vi "Dashboard Main bad.vi"() -> ()   [LabVIEW 2012]
uses:
  <vilib>/event_ctls.llb/eventvkey.ctl
  <vilib>/Utility/config.llb/Read Key (String).vi
  <vilib>/Utility/config.llb/Read Key (I32).vi
  <vilib>/Utility/config.llb/Write Key (String).vi
  <vilib>/Utility/config.llb/Write Key (I32).vi
  Program Files (x86)/National Instruments/LabVIEW 2012/examples/FRC/Vision/Rectangular Target - 2013/Robot Global Data.vi
  <vilib>/Utility/config.llb/NI_LVConfig.lvlib
  <vilib>/vision/NI_Vision_Development_Module.lvlib
  <vilib>/gmath/NI_Gmath.lvlib
panel:
  out "mean red":dbl
  out "mean blue":dbl
  out "mean green":dbl
  out "max red":dbl
  out "min red":dbl
  out "max blue":dbl
  out "min blue":dbl
  out "max green":dbl
  out "min green":dbl
  in  "Margins":cluster{"Hue":i32, "Sat":i32, "Val":i32}={"Hue"=33, "Sat"=53, "Val"=9} {"Sat" scale=0.0..80.0; "Val" scale=0.0..80.0; "Hue" scale=0.0..80.0}
  in  "Hue 2":i32(knob)=65 scale=0.0..255.0
  in  "Saturation 2":i32=255
  in  "Luminance":i32=255
  out "Hue":cluster{i32, i32}
  out "Saturation":cluster{i32, i32}
  out "Value":cluster{i32, i32}
  out "Target Info":T1(array[cluster])
  in  "Score Limits":T2={"Rect Coverage"=60.0, "X Edge Strength"=40.0, "Y Edge Strength"=60.0, "Center"=75.0, "Outer"=75.0}
  in  "Area Size Limit %":dbl=0.5
  in  "Particle Count Limit":i32=8
  out "Battery Value":dbl(slide) scale=0.0..14.0 scale format="%#_2e"
  out "Battery":sgl(graph)
  in  "Camera Settings":T3={"Frate Rate"=30, "Compression"=30, "Size"=1} {"Frate Rate" scale=1.0..30.0; "Size" items=["640x480", "320x240", "160x120"]}
  out "Mode":T4(ring)=enum."Auto Disabled"
  out "Camera IP":string
  out "JS1 Z":dbl(slide) scale=-1.0..1.0 scale format="%#_2e"
  out "JS2 Z":dbl(slide) scale=-1.0..1.0 scale format="%#_2e"
  out "Joystick 1":cluster{"X":dbl, "Y":dbl}[](graph)
  out "Joystick 2":cluster{"X":dbl, "Y":dbl}[](graph)
  out "JS Buttons 1":T5
  out "JS Buttons 2":T5
  out "MotorSlide4":dbl(slide) scale=-1.0..1.0 scale format="%#_2e"
  out "MotorSlide3":dbl(slide) scale=-1.0..1.0 scale format="%#_2e"
  out "MotorSlide2":dbl(slide) scale=-1.0..1.0 scale format="%#_2e"
  in  "MotorName3":string="Front Left"
  in  "MotorName4":string="Front Right"
  in  "MotorName1":string="Rear Left"
  in  "MotorName2":string="Rear Right"
  out "MotorChart4":dbl(graph)
  out "MotorChart3":dbl(graph)
  out "MotorChart2":dbl(graph)
  out "MotorSlide1":dbl(slide) scale=-1.0..1.0 scale format="%#_2e"
  out "MotorChart1":dbl(graph)
  out "Robot IP":string
  in  "Dashboard Tab":enum32{"Operation", "Test", "Checklist"}(tab)
  in  "Checkbox 2":bool
  in  "Checkbox 1":bool
  in  "Slider 1":dbl(slide) scale=0.0..100.0
  in  "Slider":dbl(slide) scale=0.0..100.0 scale format="%#_3g"
  in  "On/Off":bool caption="Solenoid"
  in  "Test Name":u16(ring) items=["Select the test to run...", "Example Test", "-------------------------------", "List of tests is built in robot code.", "Replace with your own automated tests."]
  in  "Test Tree":string(tree)
  in  "Motor":cluster{"Value":dbl, "Enable":bool} {"Value" scale=-1.0..1.0 scale format="%#_3g"}
  out "Progress":T6 {"Test Progress" scale=0.0..100.0}
  in  "Rev/Fwd":cluster{"Forward":bool, "Reverse":bool}
  in  "Ring":u16(ring) items=["Auto", "Fixed indoor", "Fixed outdoor 1", "Fixed outdoor 2", "Fixed fluorescent 1", "Fixed fluorescent 2", "Hold current"]
  in  "Listbox":i32(listbox)
  in  "Viewer":T7(tab)
  out "Mbps":dbl format="%#.1g"
  in  "Enable":bool=TRUE
  in  "DB Camera Config":bool
  out "Mbps":bool
  out "fps":dbl format="%#.1g"
  out "Image Error Message":string="Timeout in Camera Communications"
  out "Original Image":T8(plugin-control)
  in  "View":bool=TRUE
  out "Processed Image":T8(plugin-control)
  in  "View 2":bool=TRUE
  out "Tree":string(tree)
  # "Drive & Motors"
  # "Robot IP:"
  # "Customize by placing controls and indicators here and name to match\nDashboard Variables on robot."
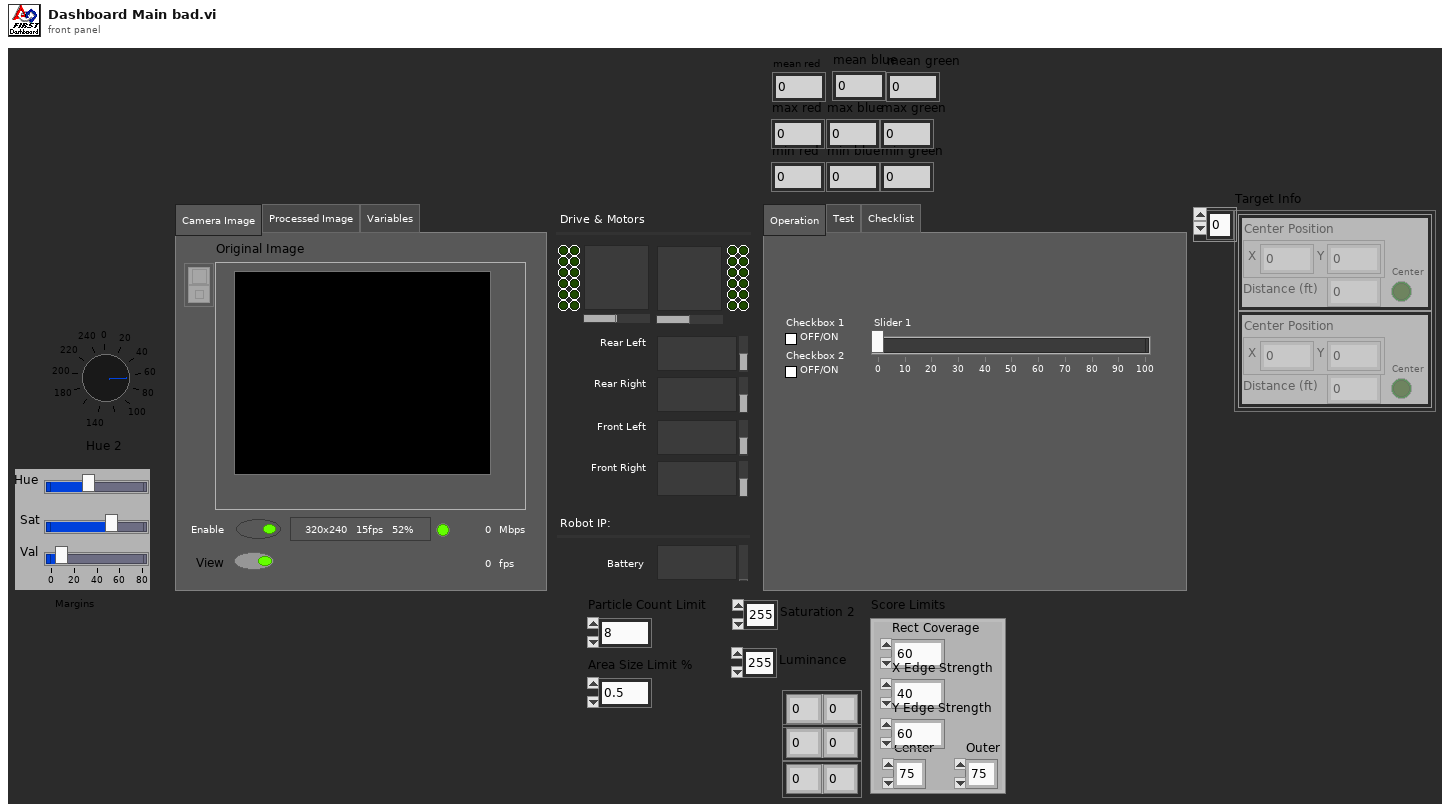
[diagram p1: front panel]
types:
  T1 = cluster{"Center Position":cluster{"X":dbl, "Y":dbl}, "Distance (ft)":dbl, "Center":bool}[]
  T2 = cluster{"Rect Coverage":dbl, "X Edge Strength":dbl, "Y Edge Strength":dbl, "Center":dbl, "Outer":dbl}
  T3 = cluster{"Frate Rate":i32, "Compression":i32, "Size":u16}
  T4 = enum8{"Tele-Op Disabled", "Tele-Op Enabled", "Auto Disabled", "Auto Enabled", "Test Disabled", "Test Enabled", ""}
  T5 = cluster{bool, bool, bool, bool, bool, bool, bool, bool, bool, bool, bool, bool}
  T6 = cluster{"Test Progress":u8, "Test Progress Text":string}
  T7 = enum32{"Camera Image", "Processed Image", "Variables"}
  T8 = typedef "IMAQ Image.ctl" = refnum<image>
  T9 = typedef "Image Type" = u32
  T10 = typedef "LVRectTypeDef.ctl" = cluster{"Left":i16, "Top":i16, "Right":i16, "Bottom":i16}
  T11 = cluster{"Left":i16, "Top":i16, "Right":i16, "Bottom":i16}
  T12 = cluster{"Competition mode":bool, "Robot Link":bool, "Autonomous":bool, "Enabled":bool, "E-Stop":bool, "Simulated":bool, "TestMode":bool, "Docked Window":bool}
  T13 = cluster{"Boolean Array[0]":bool, "Boolean Array[1]":bool, "Boolean Array[2]":bool, "Boolean Array[3]":bool, "Boolean Array[4]":bool, "Boolean Array[5]":bool, "Boolean Array[6]":bool, "Boolean Array[7]":bool, "Boolean Array[8]":bool, "Boolean Array[9]":bool, "Boolean Array[10]":bool, "Boolean Array[11]":bool}
  T14 = cluster{"Position":cluster{"X":dbl, "Y":dbl}, "Distance (ft)":dbl, "Center":bool}[]
  T15 = enum16{"arithmetic", "geometric", "harmonic", "trimmed", "median"}
  T16 = cluster{cluster{"Left":dbl, "Top":dbl, "Right":dbl, "Bottom":dbl}, "Scores":dbl[], cluster{"Long":dbl, "Short":dbl}}[]
  T17 = cluster{"Target Center (-1 to 1)":cluster{"X":dbl, "Y":dbl}, "Distance (ft)":dbl, "Center Target":bool}
  T18 = cluster{"Target Center (-1 to 1)":cluster{"X":dbl, "Y":dbl}, "Distance (ft)":dbl, "Center Target":bool}[]
  T19 = cluster{"Left":dbl, "Top":dbl, "Right":dbl, "Bottom":dbl}
  T20 = typedef "NI_LVConfig.lvlib/Config Data RefNum.ctl" = refnum<k1>
  T21 = typedef "eventvkey.ctl" = enum16{"ASCII", "Enter", "Return", "Shift", "Ctrl", "Alt", "Cmd", "Opt", "Caps", "NumLock", "Clear", "Break", "Up", "Down", "Left", "Right", "Insert", "Delete", "Home", "End", "PageUp", "PageDown", "Escape", "Help", "Pause", "ScrollLock", "F1", "F2", "F3", "F4", "F5", "F6", "F7", "F8", "F9", "F10", "F11", "F12", "F13", "F14", "F15", "F16", "F17", "F18", "F19", "F20", "F21", "F22", "F23", "F24", "Play", "VolumeUp", "VolumeDown", "Mute", "Two Byte Char"}
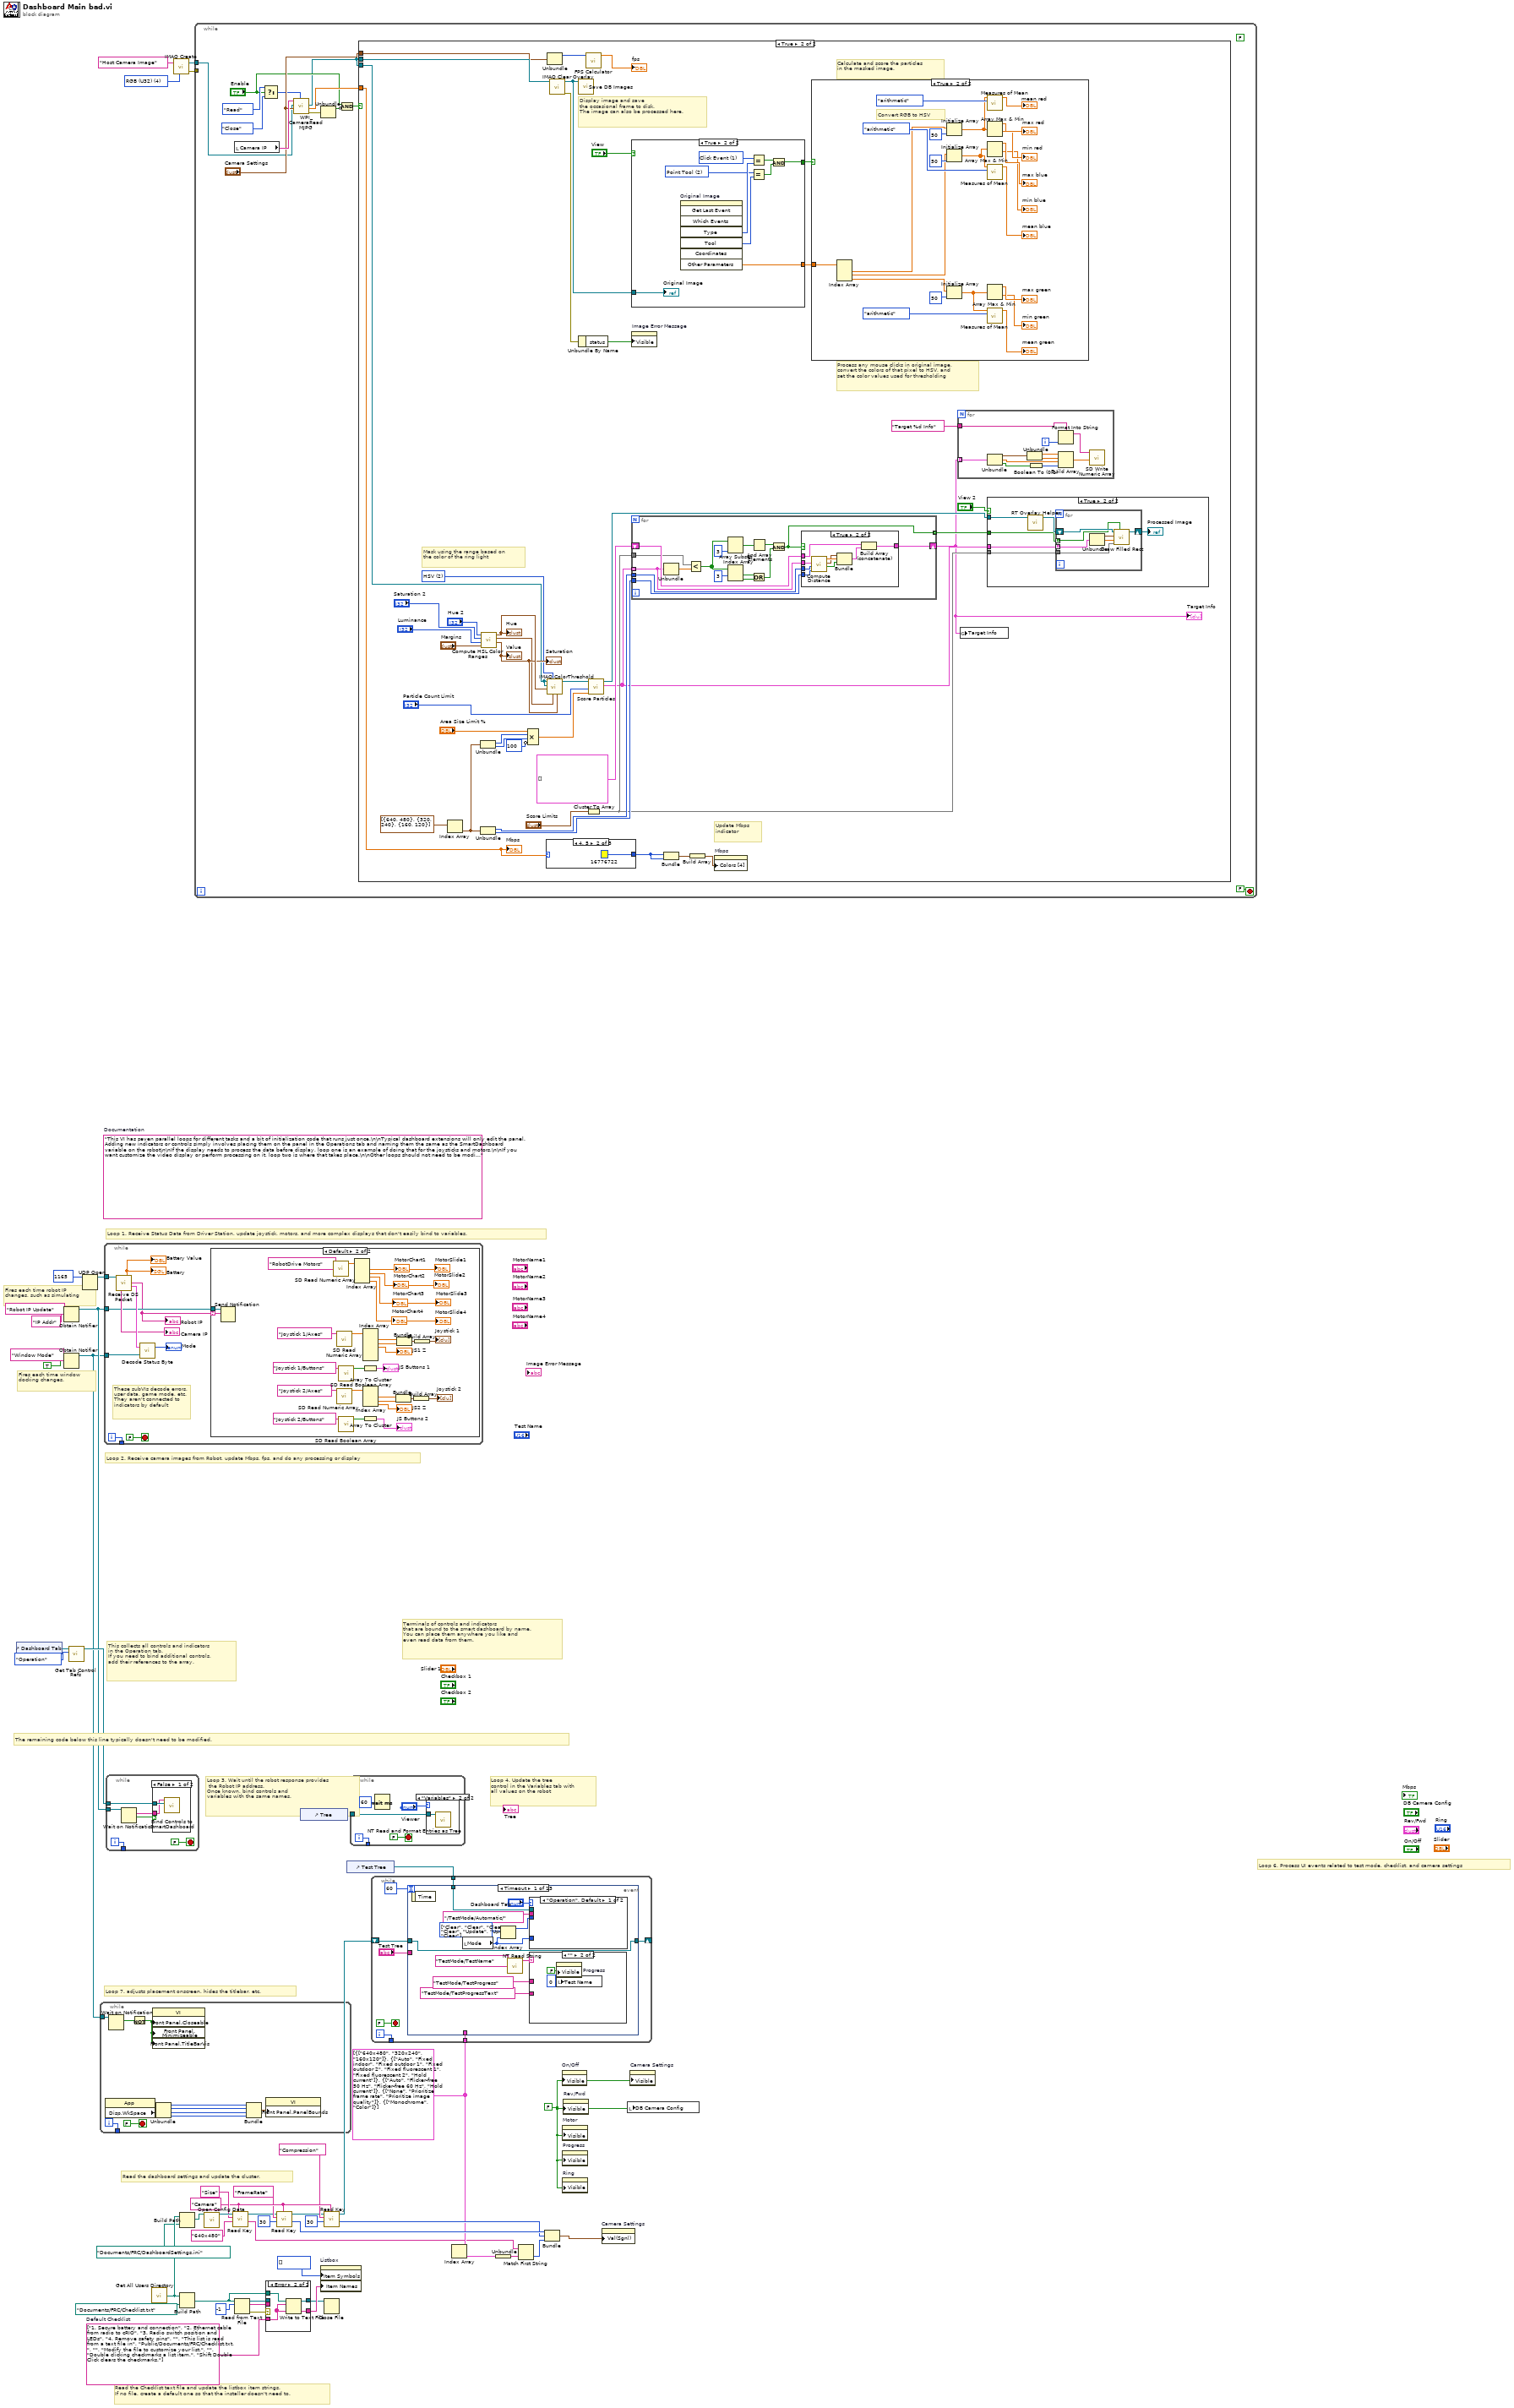
[diagram p0: block diagram]
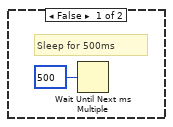
[diagram p3: hidden frame]
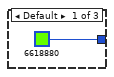
[diagram p8: hidden frame]
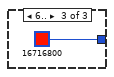
[diagram p9: hidden frame]
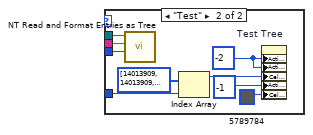
[diagram p11: hidden frame]
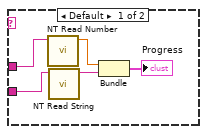
[diagram p12: hidden frame]
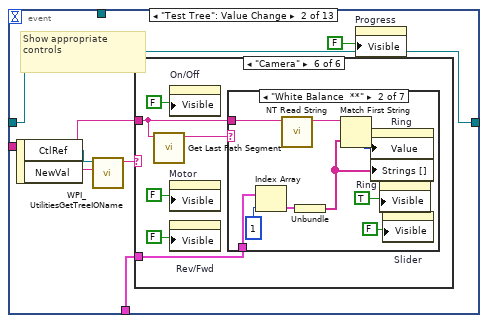
[diagram p13: hidden frame]
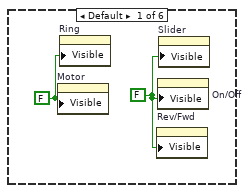
[diagram p14: hidden frame]
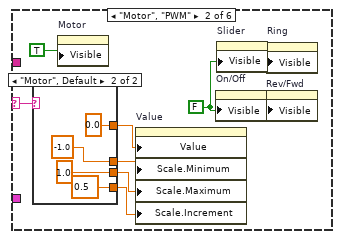
[diagram p15: hidden frame]
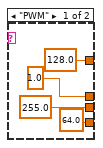
[diagram p16: hidden frame]
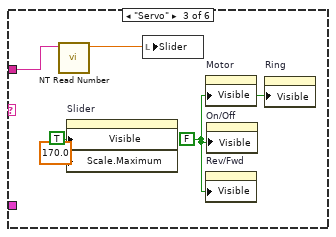
[diagram p17: hidden frame]
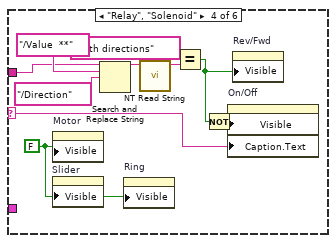
[diagram p18: hidden frame]
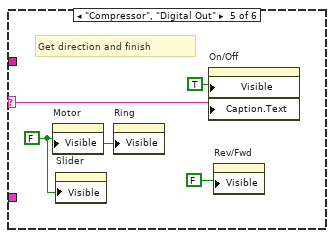
[diagram p19: hidden frame]
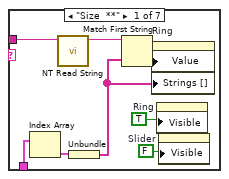
[diagram p20: hidden frame]
diagram:
  w21 = "Camera"
  w13 = cluster{string[]}[] [{["640x480", "320x240", "160x120"]}, {["Auto", "Fixed indoor", "Fixed outdoor 1", "Fixed outdoor 2", "Fixed fluorescent 1", "Fixed fluorescent 2", "Hold current"]}, {["Auto", "Flicker-free 50 Hz", "Flicker-free 60 Hz", "Hold current"]}, {["None", "Prioritize frame rate", "Prioritize image quality"]}, {["Monochrome", "Color"]}]
  w29 = string[] ["1. Secure battery and connection", "2. Ethernet cable from radio to cRIO", "3. Radio switch position and LEDs", "4. Remove safety pins", "", "This list is read from a text file in", "Public/Documents/FRC/Checklist.txt.", "", "Modify the file to customize your list.", "", "Double clicking checkmarks a list item.", "Shift Double Click clears the checkmarks."]  # Default Checklist
  w27 = FALSE ("Visible")
  (unwired) "This VI has seven parallel loops for different tasks and a bit of initialization code that runs just once.\n\nTypical dashboard extensions will only edit the panel. Adding new indicators or controls simply involves placing them on the panel in the Operations tab and naming them the same as the SmartDashboard variable on the robot\n\nIf the display needs to process the data before display, loop one is an example of doing that for the joysticks and motors.\n\nIf you want customize the video display or perform processing on it, loop two is where that takes place.\n\nOther loops should not need to be modified. They are pretty standard, and document the task they perform."  # Documentation
  w48 = T9 4 items=["Grayscale (U8)", "Grayscale (I16)", "Grayscale (SGL)", "Complex (CSG)", "RGB (U32)", "HSL (U32)", "RGB (U64)"] ("Image Type")
  # "Fires each time robot IP\nchanges, such as simulating"
  # "Fires each time window\ndocking changes."
  # "Read the Checklist text file and update the listbox item strings.\nIf no file, create a default one so that the installer doesn't need to."
  # "This collects all controls and indicators\nin the Operation tab.\nIf you need to bind additional controls,\nadd their references to the array."
  # "The remaining code below this line typically doesn't need to be modified."
  # "Loop 6. Process UI events related to test mode, checklist, and camera settings"
  # "Read the dashboard settings and update the cluster."
  # "Terminals of controls and indicators\nthat are bound to the smart dashboard by name.\nYou can place them anywhere you like and\neven read data from them."
  # "Loop 4. Update the tree\ncontrol in the Variables tab with\nall values on the robot"
  # "Loop 3. Wait until the robot response provides\n the Robot IP address.\nOnce known, bind controls and\nvariables with the same names."
  # "Loop 7. adjusts placement onscreen, hides the titlebar, etc."
  # "Loop 1. Receive Status Data from Driver Station, update joystick, motors, and more complex displays that don't easily bind to variables."
  # "Loop 2. Receive camera images from Robot, update Mbps, fps, and do any processing or display"
  n1 = control-ref of="Dashboard Tab"() -> (w43:refnum<vi>)
  n2 = Obtain Notifier(name (unnamed)="Robot IP Update", notification data type="IP Addr" ("name (unnamed)")) -> (notifier out=w40:refnum<notifier>)  [unwired: 2 in, 2 out]
  n3 = Obtain Notifier(name (unnamed)="Window Mode", notification data type=TRUE) -> (notifier out=w33:refnum<notifier>)  [unwired: 2 in, 2 out]
  n4 = call <vilib>:"Get Tab Control Refs.vi"("Page Index"=enum32{"Operation", "Test"}."Operation" ("Dashboard Tab"), "TabControl in"=w43) -> ("ControlsOnPage"=w44:refnum<vi>[])  [unwired: 9 in]
  n5 = UDP Open(11:u16 1165 ("port")) -> (port=w49:refnum<k16>)  [unwired: 2 in, 4 out]
  n6 = while {
    tunnel: w33 -> [w60]
    tunnel: [w58] -> _
    i -> [w58]
    stop <- FALSE stop-if-true
    n7 = property class="App"() -> ("Disp.WkSpace"=w57:T10)  [unwired: 2 in, 2 out]
    n8 = Wait on Notification(notifier=w60) -> (notification=w56:bool)  [unwired: 3 in, 3 out]
    n9 = Not(x=w56) -> (.not. x?=w59:bool)
    n10 = property class="VI"("Front Panel.Closeable"=w59, "Front Panel.Minimizeable"=w59, "Front Panel.TitleBarVis"=w59) -> ()  [unwired: 2 in, 2 out]
    n11 = Unbundle(w57) -> ("Left"=w55:i16, "Top"=w54:i16, "Right"=w53:i16, "Bottom"=w52:i16)
    n12 = Bundle("Left"=w55, "Top"=w54, "Right"=w53, "Bottom"=w52) -> (w51:T11)  [unwired: 1 out]
    n13 = property class="VI"("Front Panel.PanelBounds"=w51) -> ()  [unwired: 2 in, 2 out]
  }
  n14 = while {
    tunnel: w49 -> [w69]
    tunnel: w40 -> [w63]
    tunnel: w33 -> [w67]
    tunnel: [w64] -> _
    i -> [w64]
    stop <- FALSE stop-if-true
    # "These subVIs decode errors, user data, game mode, etc.\nThey aren't connected to indicators by default"
    n15 = call "Receive DS Packet.vi"("Recv Socket"=w69) -> ("Battery"=→"Battery" →"Battery Value":sgl, "Robot IP Address"=w62:string, "Status"=w70:T12, "Camera IP Address"=→"Camera IP":string)  [unwired: 1 in, 10 out]
    "Robot IP" <- w62
    n16 = call "Decode Status Byte.vi"("Window Mode Notifier"=w67, "Status"=w70) -> ("Mode"=→"Mode":T4)  [unwired: 1 out]
    n17 = case shown="Default" w62 {
      selector: w62 -> [_ w72]
      tunnel: w63 -> [_ w73]
      frame "0.0.0.0" {
        # "Robot not responding, don't poll the variables"
      }
      frame Default {
        n18 = Send Notification(notification=w72, notifier=w73) -> ()  [unwired: 1 in, 2 out]
        n19 = call <vilib>:"SD Read Numeric Array.vi"("Name"="RobotDrive Motors") -> ("Numeric Array"=w96:dbl[])  [unwired: 8 in, 2 out]
        n20 = call <vilib>:"SD Read Numeric Array.vi"("Name"="Joystick 1/Axes") -> ("Numeric Array"=w89:dbl[])  [unwired: 8 in, 2 out]
        n21 = call <vilib>:"SD Read Numeric Array.vi"("Name"="Joystick 2/Axes") -> ("Numeric Array"=w83:dbl[])  [unwired: 8 in, 2 out]
        n22 = call <vilib>:"SD Read Boolean Array.vi"("Name"="Joystick 1/Buttons") -> ("Boolean Array"=w91:bool[])  [unwired: 8 in, 2 out]
        n23 = call <vilib>:"SD Read Boolean Array.vi"("Name"="Joystick 2/Buttons") -> ("Boolean Array"=w82:bool[])  [unwired: 8 in, 2 out]
        n24 = Index Array(array=w96) -> (element #1=→"MotorChart1" →"MotorSlide1":dbl, element #2=→"MotorSlide2" →"MotorChart2":dbl, element #3=→"MotorChart3" →"MotorSlide3":dbl, element #4=→"MotorChart4" →"MotorSlide4":dbl)  [unwired: 4 in]
        n25 = Array To Cluster(array=w91) -> (cluster=→"JS Buttons 1":T13)
        n26 = Array To Cluster(array=w82) -> (cluster=→"JS Buttons 2":T13)
        n27 = Index Array(array=w89) -> (element #1=w86:dbl, element #2=w87:dbl, element #3=→"JS1 Z":dbl)  [unwired: 6 in, 3 out]
        n28 = Index Array(array=w83) -> (element #1=w78:dbl, element #2=w77:dbl, element #3=→"JS2 Z":dbl)  [unwired: 3 in]
        n29 = Bundle("Numeric"=w78, "Numeric"=w77) -> (w79:cluster{"Numeric":dbl, "Numeric":dbl})  [unwired: 1 in]
        n30 = Bundle("Numeric"=w86, "Numeric"=w87) -> (w85:cluster{"Numeric":dbl, "Numeric":dbl})  [unwired: 1 in]
        n31 = Build Array(w79) -> (→"Joystick 2":cluster{"Numeric":dbl, "Numeric":dbl}[])
        n32 = Build Array(w85) -> (→"Joystick 1":cluster{"Numeric":dbl, "Numeric":dbl}[])
      }
    }
  }
  n33 = while {
    tunnel: w44 -> [w105]
    tunnel: w40 -> [w102]
    tunnel: [w100] -> _
    i -> [w100]
    stop <- FALSE stop-if-true
    n34 = Wait on Notification(notifier=w102) -> (notification=w101:string, timed out?=w103:bool)  [unwired: 3 in, 2 out]
    n35 = case shown="False" w103 {
      tunnel: w105 -> [w107 _]
      tunnel: w101 -> [w106 _]
      frame False {
        n36 = call <vilib>:"Bind Controls to SmartDashboard.vi"("Bound Control Refs"=w107, "Server IP Address"=w106) -> ()  [unwired: 10 in]
      }
      frame True {
      }
    }
  }
  n37 = call "Get All Users Directory.vi"() -> ("All User Path"=w26:path)
  n38 = call "IMAQ Create"("Image Name"="Host Camera Image", "Image Type"=w48) -> ("New Image"=w46:T8, "error out"=w45:errorcluster)  [unwired: 2 in, 1 out]
  n39 = Build Path(base path=w26, name or relative path=path "Documents/FRC/DashboardSettings.ini") -> (appended path=w25:path)
  n40 = Build Path(base path=w26, name or relative path=path "Documents/FRC/Checklist.txt") -> (appended path=w30:path)
  n41 = while {
    tunnel: w46 -> [w118]
    tunnel: w45 -> [_]
    stop <- FALSE stop-if-true
    (unwired) FALSE
    n42 = local read "Camera IP"() -> (w120:string)
    n43 = Select(t=enum16{"Read", "Reopen", "Close"}."Read" ("Operation"), s="Enable", f=enum16{"Read", "Reopen", "Close"}."Close" ("Operation")) -> (s? t:f=w114:enum16{"Read", "Reopen", "Close"})
    n44 = call <vilib>:"WPI_CameraRead MJPG.vi"("Operation"=w114, "Camera Settings"="Camera Settings", "Image"=w118, "address"=w120) -> ("error out"=w113:errorcluster, "Bandwidth (kbps)"=w117:dbl, "Image Out"=w109:T8)  [unwired: 5 in]
    n45 = Unbundle(w113) -> ("status"=w111:bool)  [unwired: 2 out]
    n46 = Compound Arithmetic op=AND("Enable", invert w111) -> (w110:bool)
    n47 = case shown="True" w110 {
      tunnel: "Camera Settings" -> [_ w156]
      tunnel: w109 -> [_ w159]
      tunnel: w117 -> [_ w158]
      tunnel: w109 -> [_ w122]
      frame False {
        # "Sleep for 500ms"
        n48 = Wait Until Next ms Multiple(millisecond multiple=u32 500) -> ()  [unwired: 1 out]
      }
      frame True {
        w129 = u16 2 items=["RGB", "HSL", "HSV", "HSI"] ("Color Mode")
        # "Mask using the range based on\nthe color of the ring light"
        # "Process any mouse clicks in original image,\nconvert the colors of that pixel to HSV, and\nset the color values used for thresholding"
        # "Calculate and score the particles\nin the masked image."
        # "Display image and save\nthe occasional frame to disk.\nThe image can also be processed here."
        # "Update Mbps\nindicator"
        n49 = Index Array(array=cluster{i32, i32}[] [{640, 480}, {320, 240}, {160, 120}]) -> (element=w123:cluster{i32, i32})  [unwired: 1 in]
        n50 = Unbundle(w123) -> (w151:i32, w152:i32)
        n51 = Unbundle(w123) -> (w146:i32, w147:i32)
        n52 = call "Compute HSL Color Ranges.vi"("Margins"="Margins", "Luminance"="Luminance", "Saturation"="Saturation 2", "Hue"="Hue 2") -> ("Lum Range"=w135:cluster{i32, i32}, "Sat Range"=w130:cluster{i32, i32}, "Hue Range"=w136:cluster{i32, i32})  [unwired: 5 in]
        "Hue" <- w136
        "Saturation" <- w135
        "Value" <- w135
        n53 = Compound Arithmetic op=MULTIPLY("Area Size Limit %", w151, w152, invert 100 ("length")) -> (w154:dbl)
        n54 = case shown="4, 5" w158 {
          tunnel: [u32 6618880 ("Color Box") u32 16776722 ("Color Box") u32 16716800 ("Color Box")] -> w160
          frame Default {
          }
          frame 4, 5 {
          }
          frame 6.. {
          }
        }
        n55 = call "IMAQ ColorThreshold"("Blue or Luma or Val or Inten Range"=w135, "Green or Sat Range"=w130, "Color Mode"=w129, "Red or Hue Range"=w136, "Image Dst"=w122, "Image Src"=w122) -> ("Image Dst Out"=w128:T8)  [unwired: 4 in, 1 out]
        n56 = Unbundle(w156) -> ("Frate Rate"=w155:i32)  [unwired: 2 out]
        n57 = call "IMAQ Clear Overlay"("Image"=w159) -> ("error out"=w163:errorcluster, "Image Out"=w137:T8)  [unwired: 2 in, 7 out]
        n58 = call "Save DB Images.vi"("Image"=w137) -> ()  [unwired: 2 in, 1 out]
        n59 = Unbundle By Name(w163) -> ("status"=w164:bool)
        n60 = call "FPS Calculator.vi"("Average Count"=w155) -> ("fps"=→"fps":dbl)  [unwired: 10 in]
        n61 = Cluster To Array(cluster="Score Limits") -> (array=w142:dbl[])
        n62 = call "Score Particles.vi"("Area Size Limit"=w154, "Particle Count Limit"="Particle Count Limit", "Image Refnum in"=w128) -> ("Scored Particle Info"=w140:T16, "Image Refnum out"=w138:T8)  [unwired: 7 in]
        n63 = case shown="True" "View" {
          tunnel: [_ w215] -> w144
          tunnel: [_ w212] -> w145
          tunnel: w137 -> [_ w211]
          frame False {
          }
          frame True {
            w213 = 2 items=["None", "Selection Tool", "Point Tool", "Line Tool", "Rectangle Tool", "Oval Tool", "Polygon Tool", "ClosedFreehandTool", "Annulus Tool", "Rotated Rectangle Tool", "Zoom Tool", "Pan Tool", "Polyline Tool", "Freehand Tool"] ("Tool")
            w214 = 1 items=["No Event"=0, "Click Event"=1, "Draw Event"=2, "Size Event"=4, "Scroll Event"=5, "Double Click Event"=8] ("Type")
            n64 = invoke on="Original Image" class="ImageControl" method="Get Last Event"() -> ("Type"=w216:i32, "Tool"=w219:i32, "Other Parameters"=w212:sgl[])  [unwired: 8 in, 5 out]
            n65 = Equal?(x=w214, y=w216) -> (x = y?=w217:bool)
            n66 = Equal?(x=w213, y=w219) -> (x = y?=w218:bool)
            n67 = And(x=w217, y=w218) -> (x .and. y?=w215:bool)
            "Original Image" <- w211
          }
        }
        n68 = property on="Image Error Message" class="Str"("Visible"=w164) -> ()  [unwired: 2 in, 2 out]
        n69 = for {
          shift-right: [w234] -> w126
          shift-left: T14 [] -> [w235]
          tunnel: w146 -> [w233]
          tunnel: w140 -> [w229] mode=indexing
          tunnel: w142 -> [w231]
          tunnel: w147 -> [w230]
          tunnel: [w220] -> w149 mode=indexing
          n70 = Unbundle(w229) -> ("Scores"=w232:dbl[])  [unwired: 2 out]
          n71 = Less?(x=w231, y=w232) -> (x < y?=w221:bool[])
          n72 = Array Subset(array=w221, length=3) -> (w223:bool[])  [unwired: 1 in]
          n73 = Index Array(array=w221, index #1=3 ("length")) -> (element #1=w225:bool, element #2=w226:bool)  [unwired: 1 in]
          n74 = Or(x=w225, y=w226) -> (x .or. y?=w227:bool)
          n75 = And Array Elements(Boolean array=w223) -> (logical AND=w228:bool)
          n76 = And(x=w228, y=w227) -> (x .and. y?=w220:bool)
          n77 = case shown="True" w220 {
            tunnel: w235 -> [w236 w245]
            tunnel: [w236 w244] -> w234
            tunnel: w233 -> [_ w242]
            tunnel: w230 -> [_ w240]
            tunnel: w229 -> [_ w238]
            frame False {
            }
            frame True {
              n78 = call "Compute Distance.vi"("Y Image Resolution"=w240, "X Image Resolution"=w242, "Particle Scores"=w238) -> ("Center Target"=w237:bool, "Target Center (-1 to 1)"=w239:cluster{"X":dbl, "Y":dbl}, "Distance (ft)"=w241:dbl)  [unwired: 6 in]
              n79 = Bundle("Target Center (-1 to 1)"=w239, "Distance (ft)"=w241, "Center Target"=w237) -> (w243:T17)  [unwired: 1 in]
              n80 = Build Array (concatenate)(w245, w243) -> (w244:T18)
            }
          }
        }
        "Target Info" <- w126
        n81 = Bundle("Color Box"=w160, "Color Box"=w160) -> (w162:cluster{"Color Box":u32, "Color Box":u32})  [unwired: 1 out]
        n82 = Build Array(w162) -> (w161:cluster{"Color Box":u32, "Color Box":u32}[])
        n83 = property on="Mbps" class="Bool (strict)"("Colors [4]"=w161) -> ()  [unwired: 2 in, 2 out]
        n84 = case shown="True" w144 {
          tunnel: w145 -> [_ w197]
          frame False {
          }
          frame True {
            # "Convert RGB to HSV"
            n85 = Index Array(array=w197) -> (element #1=w187:sgl, element #2=w186:sgl, element #3=w185:sgl)  [unwired: 3 in]
            n86 = Initialize Array(w187, 50 ("dimension size")) -> (w184:sgl[])
            n87 = Initialize Array(w186, 50 ("dimension size")) -> (w181:sgl[])
            n88 = Initialize Array(w185, 50 ("dimension size")) -> (w176:sgl[])
            n89 = call <vilib>:"Measures of Mean.vi"("type"=T15."arithmetic", "x array"=w184) -> ("mean value"=→"mean red":dbl)  [unwired: 8 in, 1 out]
            n90 = Array Max & Min(array=w184) -> (max value=→"max red":sgl, min value=→"min red":sgl)  [unwired: 2 out]
            n91 = Array Max & Min(array=w181) -> (max value=→"max blue":sgl, min value=→"min blue":sgl)  [unwired: 2 out]
            n92 = call <vilib>:"Measures of Mean.vi"("type"=T15."arithmetic", "x array"=w181) -> ("mean value"=→"mean blue":dbl)  [unwired: 8 in, 1 out]
            n93 = Array Max & Min(array=w176) -> (max value=→"max green":sgl, min value=→"min green":sgl)  [unwired: 2 out]
            n94 = call <vilib>:"Measures of Mean.vi"("type"=T15."arithmetic", "x array"=w176) -> ("mean value"=→"mean green":dbl)  [unwired: 8 in, 1 out]
          }
        }
        n95 = for {
          tunnel: "Target %d Info" ("Name") -> [w167]
          tunnel: w126 -> [w166] mode=indexing
          i -> [w165]
          n96 = Unbundle(w166) -> ("Position"=w169:cluster{"X":dbl, "Y":dbl}, "Distance (ft)"=w173:dbl, "Center"=w170:bool)
          n97 = Unbundle(w169) -> ("X"=w171:dbl, "Y"=w172:dbl)
          n98 = Boolean To (0,1)(Boolean=w170) -> (0, 1=w174:i16)
          n99 = Format Into String(format string=w167, w165) -> (resulting string=w168:string)  [unwired: 2 in, 1 out]
          n100 = Build Array(w171, w172, w173, w174) -> (w175:dbl[])
          n101 = call <vilib>:"SD Write Numeric Array.vi"("Numeric Array"=w175, "Name"=w168) -> ()  [unwired: 8 in, 2 out]
        }
        n102 = global write "Robot Global Data.vi" "Target Info"(w126) -> ()
        n103 = case shown="True" "View 2" {
          tunnel: w138 -> [_ w200]
          tunnel: w140 -> [_ w202]
          tunnel: w142 -> [_ w201]
          tunnel: w149 -> [_ w198]
          frame False {
          }
          frame True {
            n104 = call "RT Overlay Helper.vi"("Refnum in"=w200) -> ("Refnum out"=w203:T8)  [unwired: 10 in]
            n105 = for {
              shift-right: [w209] -> w199
              shift-left: w203 -> [w210]
              tunnel: w202 -> [w206] mode=indexing
              tunnel: w201 -> [w205]
              tunnel: w198 -> [w204] mode=indexing
              n106 = Unbundle(w206) -> (w207:T19, "Scores"=w208:dbl[])  [unwired: 1 out]
              n107 = call "Draw Filled Rect.vi"("Limit Passed"=w204, "Limits"=w205, "Scores"=w208, "Bounding Box"=w207, "image in"=w210) -> ("image out"=w209:T8)  [unwired: 6 in]
            }
            "Processed Image" <- w199
          }
        }
        "Mbps" <- w158
      }
    }
  }
  n108 = call <vilib>:"Open Config Data.vi"("configuration file path"=w25) -> ("refnum"=w24:T20)  [unwired: 8 in, 2 out]
  n109 = call-poly <vilib>:"Read Key.vi"("section"=w21, "default value"="640x480", "key"="Size", "refnum"=w24) -> ("value"=w11:string, "refnum out"=w6:T20)  [unwired: 2 in, 4 out]
  n110 = Read from Text File(file (use dialog)=w30, count=-1 ("timeout ms (25000)")) -> (refnum out=w8:refnum<file>, text=w31:string[], error out=w32:errorcluster)  [unwired: 2 in, 1 out]
  n111 = case shown="Error" w32 {
    tunnel: w31 -> [w250 _]
    tunnel: [w250 w252] -> w28
    tunnel: w29 -> [_ w252]
    tunnel: w30 -> [_ w253]
    tunnel: [w249 w251] -> w7
    tunnel: w8 -> [w249 _]
    frame No Error {
    }
    frame Error {
      n112 = Write to Text File(file (use dialog)=w253, text=w252) -> (refnum out=w251:refnum<file>)  [unwired: 2 in, 2 out]
    }
  }
  n113 = call-poly <vilib>:"Read Key.vi"("section"=w21, "default value"=30, "key"="FrameRate", "refnum"=w6) -> ("value"=w16:i32, "refnum out"=w5:T20)  [unwired: 1 in, 5 out]
  n114 = control-ref of="Tree"() -> (w2:refnum<vi>)
  n115 = property on="Listbox" class="LstBox (strict)"("Item Symbols"=i32[] [], "Item Names"=w28) -> ()  [unwired: 2 in, 2 out]
  n116 = Close File(refnum=w7) -> ()  [unwired: 1 in, 2 out]
  n117 = call-poly <vilib>:"Read Key.vi"("section"=w21, "default value"=30, "key"="Compression", "refnum"=w5) -> ("value"=w15:i32, "refnum out"=w3:T20)  [unwired: 1 in, 5 out]
  n118 = control-ref of="Test Tree"() -> (w1:refnum<vi>)
  n119 = while {
    tunnel: [w255] -> _
    tunnel: w2 -> [w254]
    i -> [w255]
    stop <- FALSE stop-if-true
    n120 = Wait (ms)(milliseconds to wait=u32 60) -> ()  [unwired: 1 out]
    n121 = case shown="\"Variables\"" "Viewer" {
      tunnel: w254 -> [_ w259]
      frame Default {
      }
      frame "Variables" {
        n122 = call <vilib>:"NT Read and Format Entries as Tree.vi"("Tree Refnum"=w259) -> ()  [unwired: 9 in, 2 out]
      }
    }
  }
  n123 = while {
    tunnel: w13 -> [w264]
    shift-right: [w263] -> _
    shift-left: w3 -> [w262]
    tunnel: [w261] -> _
    tunnel: w1 -> [w260]
    i -> [w261]
    stop <- FALSE stop-if-true
    n124 = event shown="[0] Timeout" {
      selector: _ -> [_ _ _ _ _ _ _ _ _ _ _ _ _]
      dyn-events: _ -> [_ _ _ _ _ _ _ _ _ _ _ _ _]
      timeout: u32 60 ("milliseconds to wait") -> [_ _ _ _ _ _ _ _ _ _ _ _ _]
      tunnel: w260 -> [w274 _ _ _ _ _ _ _ _ _ _ _ _]
      tunnel: "Test Tree" -> [_ _ _ _ _ _ _ _ w468 w476 w478 w482 w490]
      tunnel: w264 -> [_ w296 _ _ _ _ w432 w462 _ _ _ _ _]
      tunnel: [w268 w295 _ w398 w406 w418 w431 w455 w467 w474 w477 w481 w489] -> w263
      tunnel: w262 -> [w268 w295 _ w398 w406 w418 w430 w455 w467 w474 w477 w481 w489]
      event Timeout {
        w273 = enum16{"Update", "Clear"}[] [enum."Clear", enum."Clear", enum."Clear", enum."Clear", enum."Update", enum."Update", enum."Clear"] items=["Update", "Clear"]
        n125 = event-data() -> ()  [unwired: 1 in, 1 out]
        n126 = local read "Mode"() -> (w271:T4)
        n127 = Index Array(array=w273, index=w271) -> (element=w272:enum16{"Update", "Clear"})
        n128 = call <vilib>:"NT Read String.vi"("Name"="TestMode/TestName") -> ("String"=w277:string)  [unwired: 9 in, 1 out]
        n129 = case shown="\"Operation\", Default" "Dashboard Tab" {
          tunnel: w274 -> [_ w287]
          tunnel: "/TestMode/Automatic/" ("Name Pattern") -> [_ w286]
          tunnel: w272 -> [_ w285]
          tunnel: w271 -> [_ w283]
          frame "Operation", Default {
          }
          frame "Test" {
            w282 = -2 ("Active Item:Row Number")
            n130 = call <vilib>:"NT Read and Format Entries as Tree.vi"("Operation"=w285, "Name Pattern"=w286, "Tree Refnum"=w287) -> ()  [unwired: 7 in, 2 out]
            n131 = Index Array(array=u32[] [14013909, 14013909, 14013909, 14013909, 14013909, 16777215, 14013909], index=w283) -> (element=w281:u32)
            n132 = property on="Test Tree" class="Tree (strict)"("Active Item Row Number"=w282, "ActiveColNum"=w282, "CellBG"=w281, "Active Item Row Number"=-1 ("Active Item:Row Number"), "CellBG"=u32 5789784 ("Color Box")) -> ()  [unwired: 2 in, 2 out]
          }
        }
        n133 = case shown="\"\"" w277 {
          tunnel: "TestMode/TestProgress" ("Name") -> [w289 _]
          tunnel: "TestMode/TestProgressText" ("Name") -> [w288 _]
          frame Default {
            n134 = call <vilib>:"NT Read Number.vi"("Name"=w289) -> ("Numeric"=w290:dbl)  [unwired: 9 in, 1 out]
            n135 = call <vilib>:"NT Read String.vi"("Name"=w288) -> ("String"=w291:string)  [unwired: 9 in, 1 out]
            n136 = Bundle("Numeric"=w290, "String"=w291) -> (→"Progress":cluster{"Numeric":dbl, "String":string})  [unwired: 1 in]
          }
          frame "" {
            n137 = local write "Test Name"(u16 0) -> ()
            n138 = property on="Progress" class="Clust (strict)"("Visible"=FALSE) -> ()  [unwired: 2 in, 2 out]
          }
        }
      }
      event "Test Tree": Value Change {
        # "Show appropriate\ncontrols"
        n139 = event-data() -> ("CtlRef"=w299:refnum<vi>, "NewVal"=w297:string)  [unwired: 1 in]
        n140 = call <vilib>:"WPI_UtilitiesGetTreeIOName.vi"("NewVal"=w297, "TreeControl in"=w299) -> ("I/O Name"=w300:string)  [unwired: 9 in]
        n141 = case shown="\"Camera\"" w300 {
          selector: w300 -> [_ w307 _ w325 w334 _]
          tunnel: w297 -> [_ _ w322 w324 _ w341]
          tunnel: w296 -> [_ _ _ _ _ w340]
          frame Default {
            w302 = FALSE ("Visible")
            w301 = FALSE ("Visible")
            n142 = property on="Motor" class="Clust (strict)"("Visible"=w301) -> ()  [unwired: 2 in, 2 out]
            n143 = property on="Ring" class="Ring (strict)"("Visible"=w301) -> ()  [unwired: 2 in, 2 out]
            n144 = property on="Rev/Fwd" class="Clust (strict)"("Visible"=w302) -> ()  [unwired: 2 in, 2 out]
            n145 = property on="On/Off" class="Bool (strict)"("Visible"=w302) -> ()  [unwired: 2 in, 2 out]
            n146 = property on="Slider" class="Slide (strict)"("Visible"=w302) -> ()  [unwired: 2 in, 2 out]
          }
          frame "Motor", "PWM" {
            w308 = FALSE ("Visible")
            n147 = case shown="\"Motor\", Default" w307 {
              tunnel: [1.0 ("Value") -1.0 ("Value")] -> w306
              tunnel: [255.0 ("Value") 1.0 ("Value")] -> w305
              tunnel: [128.0 ("Value") 0.0 ("Value")] -> w304
              tunnel: [64.0 ("Value") 0.5 ("Value")] -> w303
              frame "PWM" {
              }
              frame "Motor", Default {
              }
            }
            n148 = property on="Motor" class="Clust (strict)"("Visible"=TRUE) -> ()  [unwired: 2 in, 2 out]
            n149 = property on="Value" class="Slide (strict)"("Value"=w304, "Scale.Minimum"=w306, "Scale.Maximum"=w305, "Scale.Increment"=w303) -> ()  [unwired: 2 in, 2 out]
            n150 = property on="On/Off" class="Bool (strict)"("Visible"=w308) -> ()  [unwired: 2 in, 2 out]
            n151 = property on="Slider" class="Slide (strict)"("Visible"=w308) -> ()  [unwired: 2 in, 2 out]
            n152 = property on="Ring" class="Ring (strict)"("Visible"=w308) -> ()  [unwired: 2 in, 2 out]
            n153 = property on="Rev/Fwd" class="Clust (strict)"("Visible"=w308) -> ()  [unwired: 2 in, 2 out]
          }
          frame "Servo" {
            w320 = FALSE ("Visible")
            n154 = call <vilib>:"NT Read Number.vi"("Name"=w322) -> ("Numeric"=w321:dbl)  [unwired: 9 in, 1 out]
            n155 = property on="Slider" class="Slide (strict)"("Visible"=TRUE, "Scale.Maximum"=170.0 ("Scale.Range:Maximum")) -> ()  [unwired: 2 in, 2 out]
            n156 = local write "Slider"(w321) -> ()
            n157 = property on="Motor" class="Clust (strict)"("Visible"=w320) -> ()  [unwired: 2 in, 2 out]
            n158 = property on="Rev/Fwd" class="Clust (strict)"("Visible"=w320) -> ()  [unwired: 2 in, 2 out]
            n159 = property on="On/Off" class="Bool (strict)"("Visible"=w320) -> ()  [unwired: 2 in, 2 out]
            n160 = property on="Ring" class="Ring (strict)"("Visible"=w320) -> ()  [unwired: 2 in, 2 out]
          }
          frame "Relay", "Solenoid" {
            w323 = FALSE ("Visible")
            n161 = property on="Motor" class="Clust (strict)"("Visible"=w323) -> ()  [unwired: 2 in, 2 out]
            n162 = property on="Slider" class="Slide (strict)"("Visible"=w323) -> ()  [unwired: 2 in, 2 out]
            n163 = Search and Replace String(input string=w324, search string="/Value  **", replace string="/Direction") -> (result string=w330:string)  [unwired: 5 in, 3 out]
            n164 = property on="Ring" class="Ring (strict)"("Visible"=w323) -> ()  [unwired: 2 in, 2 out]
            n165 = call <vilib>:"NT Read String.vi"("Name"=w330) -> ("String"=w328:string)  [unwired: 9 in, 1 out]
            n166 = Equal?(x="Both directions", y=w328) -> (x = y?=w326:bool)
            n167 = Not(x=w326) -> (.not. x?=w327:bool)
            n168 = property on="On/Off" class="Bool (strict)"("Visible"=w327, "Caption.Text"=w325) -> ()  [unwired: 2 in, 2 out]
            n169 = property on="Rev/Fwd" class="Clust (strict)"("Visible"=w326) -> ()  [unwired: 2 in, 2 out]
          }
          frame "Compressor", "Digital Out" {
            w333 = FALSE ("Visible")
            # "Get direction and finish"
            n170 = property on="Motor" class="Clust (strict)"("Visible"=w333) -> ()  [unwired: 2 in, 2 out]
            n171 = property on="Slider" class="Slide (strict)"("Visible"=w333) -> ()  [unwired: 2 in, 2 out]
            n172 = property on="Ring" class="Ring (strict)"("Visible"=w333) -> ()  [unwired: 2 in, 2 out]
            n173 = property on="On/Off" class="Bool (strict)"("Visible"=TRUE, "Caption.Text"=w334) -> ()  [unwired: 2 in, 2 out]
            n174 = property on="Rev/Fwd" class="Clust (strict)"("Visible"=FALSE) -> ()  [unwired: 2 in, 2 out]
          }
          frame "Camera" {
            n175 = call <vilib>:"Get Last Path Segment.vi"("String in"=w341) -> ("String out"=w342:string)  [unwired: 10 in]
            n176 = property on="On/Off" class="Bool (strict)"("Visible"=FALSE) -> ()  [unwired: 2 in, 2 out]
            n177 = property on="Motor" class="Clust (strict)"("Visible"=FALSE) -> ()  [unwired: 2 in, 2 out]
            n178 = property on="Rev/Fwd" class="Clust (strict)"("Visible"=FALSE) -> ()  [unwired: 2 in, 2 out]
            n179 = case shown="\"White Balance  **\"" w342 {
              tunnel: w341 -> [w348 w357 w366 w375 w384 _ w390]
              tunnel: w340 -> [w346 w354 w363 w372 w381 _ _]
              frame "Size  **" {
                n180 = Index Array(array=w346) -> (element=w345:cluster{string[]})  [unwired: 1 in]
                n181 = call <vilib>:"NT Read String.vi"("Name"=w348) -> ("String"=w347:string)  [unwired: 9 in, 1 out]
                n182 = Unbundle(w345) -> (w343:string[])
                n183 = Match First String(2:w343, 3:w347) -> (0:w344:i32)  [unwired: 1 out]
                n184 = property on="Ring" class="Ring (strict)"("Value"=w344, "Strings []"=w343) -> ()  [unwired: 2 in, 2 out]
                n185 = property on="Ring" class="Ring (strict)"("Visible"=TRUE) -> ()  [unwired: 2 in, 2 out]
                n186 = property on="Slider" class="Slide (strict)"("Visible"=FALSE) -> ()  [unwired: 2 in, 2 out]
              }
              frame "White Balance  **" {
                n187 = Index Array(array=w354, index=1) -> (element=w355:cluster{string[]})
                n188 = call <vilib>:"NT Read String.vi"("Name"=w357) -> ("String"=w356:string)  [unwired: 9 in, 1 out]
                n189 = Unbundle(w355) -> (w352:string[])
                n190 = Match First String(2:w352, 3:w356) -> (0:w351:i32)  [unwired: 1 out]
                n191 = property on="Ring" class="Ring (strict)"("Value"=w351, "Strings []"=w352) -> ()  [unwired: 2 in, 2 out]
                n192 = property on="Ring" class="Ring (strict)"("Visible"=TRUE) -> ()  [unwired: 2 in, 2 out]
                n193 = property on="Slider" class="Slide (strict)"("Visible"=FALSE) -> ()  [unwired: 2 in, 2 out]
              }
              frame "Exposure  **" {
                n194 = Index Array(array=w363, index=2) -> (element=w364:cluster{string[]})
                n195 = call <vilib>:"NT Read String.vi"("Name"=w366) -> ("String"=w365:string)  [unwired: 9 in, 1 out]
                n196 = Unbundle(w364) -> (w360:string[])
                n197 = Match First String(2:w360, 3:w365) -> (0:w361:i32)  [unwired: 1 out]
                n198 = property on="Ring" class="Ring (strict)"("Value"=w361, "Strings []"=w360) -> ()  [unwired: 2 in, 2 out]
                n199 = property on="Ring" class="Ring (strict)"("Visible"=TRUE) -> ()  [unwired: 2 in, 2 out]
                n200 = property on="Slider" class="Slide (strict)"("Visible"=FALSE) -> ()  [unwired: 2 in, 2 out]
              }
              frame "Exposure Priority  **" {
                n201 = Index Array(array=w372, index=3) -> (element=w373:cluster{string[]})
                n202 = call <vilib>:"NT Read String.vi"("Name"=w375) -> ("String"=w374:string)  [unwired: 9 in, 1 out]
                n203 = Unbundle(w373) -> (w369:string[])
                n204 = Match First String(2:w369, 3:w374) -> (0:w370:i32)  [unwired: 1 out]
                n205 = property on="Ring" class="Ring (strict)"("Value"=w370, "Strings []"=w369) -> ()  [unwired: 2 in, 2 out]
                n206 = property on="Ring" class="Ring (strict)"("Visible"=TRUE) -> ()  [unwired: 2 in, 2 out]
                n207 = property on="Slider" class="Slide (strict)"("Visible"=FALSE) -> ()  [unwired: 2 in, 2 out]
              }
              frame "Color Enable  **" {
                n208 = Index Array(array=w381, index=4) -> (element=w382:cluster{string[]})
                n209 = call <vilib>:"NT Read String.vi"("Name"=w384) -> ("String"=w383:string)  [unwired: 9 in, 1 out]
                n210 = Unbundle(w382) -> (w378:string[])
                n211 = Match First String(2:w378, 3:w383) -> (0:w379:i32)  [unwired: 1 out]
                n212 = property on="Ring" class="Ring (strict)"("Value"=w379, "Strings []"=w378) -> ()  [unwired: 2 in, 2 out]
                n213 = property on="Ring" class="Ring (strict)"("Visible"=TRUE) -> ()  [unwired: 2 in, 2 out]
                n214 = property on="Slider" class="Slide (strict)"("Visible"=FALSE) -> ()  [unwired: 2 in, 2 out]
              }
              frame Default {
                n215 = property on="Ring" class="Ring (strict)"("Visible"=FALSE) -> ()  [unwired: 2 in, 2 out]
                n216 = property on="Slider" class="Slide (strict)"("Visible"=FALSE) -> ()  [unwired: 2 in, 2 out]
              }
              frame "Brightness  **", "Color Level  **", "Compression  **", "FPS  **", "Sharpness  **" {
                n217 = call <vilib>:"NT Read Number.vi"("Name"=w390) -> ("Numeric"=w389:dbl)  [unwired: 9 in, 1 out]
                n218 = local write "Slider"(w389) -> ()
                n219 = property on="Slider" class="Slide (strict)"("Visible"=TRUE, "Scale.Maximum"=100.0 ("Scale.Range:Maximum")) -> ()  [unwired: 2 in, 2 out]
                n220 = property on="Ring" class="Ring (strict)"("Visible"=FALSE) -> ()  [unwired: 2 in, 2 out]
              }
            }
          }
        }
        n221 = property on="Progress" class="Clust (strict)"("Visible"=FALSE) -> ()  [unwired: 2 in, 2 out]
      }
      event "Test Name": Mouse Enter {
        # "Populate the ring with the list of tests"
        n222 = event-data() -> ()  [unwired: 1 in, 1 out]
        n223 = call <vilib>:"NT Read String Array.vi"("Name"="TestMode/TestList") -> ("String Array"=w397:string[])  [unwired: 9 in, 1 out]
        n224 = Build Array (concatenate)("Select the test to run...", w397) -> (w396:string[])
        n225 = property on="Test Name" class="Ring (strict)"("Strings []"=w396) -> ()  [unwired: 2 in, 2 out]
      }
      event "Test Name": Value Change {
        w399 = FALSE ("Visible")
        # "Tell the robot the test name to run"
        n226 = event-data() -> ("NewVal"=w403:u16)  [unwired: 1 in]
        n227 = property on="Test Name" class="Ring (strict)"() -> ("Strings []"=w404:string[])  [unwired: 2 in, 2 out]
        n228 = local write "Progress"(T6 {"Test Progress"=0, "Test Progress Text"=""} ("Progress")) -> ()
        n229 = Index Array(array=w404, index=w403) -> (element=w402:string)
        n230 = call <vilib>:"NT Write String.vi"("String"=w402, "Name"="TestMode/TestName") -> ()  [unwired: 9 in, 1 out]
        n231 = property on="Progress" class="Clust (strict)"("Visible"=TRUE) -> ()  [unwired: 2 in, 2 out]
        n232 = property on="Motor" class="Clust (strict)"("Visible"=w399) -> ()  [unwired: 2 in, 2 out]
        n233 = property on="Slider" class="Slide (strict)"("Visible"=w399) -> ()  [unwired: 2 in, 2 out]
        n234 = property on="On/Off" class="Bool (strict)"("Visible"=w399) -> ()  [unwired: 2 in, 2 out]
        n235 = property on="Rev/Fwd" class="Clust (strict)"("Visible"=w399) -> ()  [unwired: 2 in, 2 out]
        n236 = property on="Ring" class="Ring (strict)"("Visible"=w399) -> ()  [unwired: 2 in, 2 out]
      }
      event "Listbox": Double Click {
        n237 = event-data() -> ("PlatMods.Shift"=w407:bool, "Row"=w409:i32)  [unwired: 1 in]
        n238 = case shown="False" w407 {
          tunnel: w409 -> [w413 _]
          tunnel: 1 -> [w412 _]
          frame False {
            n239 = property on="Listbox" class="LstBox (strict)"() -> ("Item Symbols"=w411:i32[])  [unwired: 2 in, 2 out]
            n240 = Replace Array Subset(array=w411, new element=w412, index=w413) -> (w410:i32[])
            n241 = property on="Listbox" class="LstBox (strict)"("Item Symbols"=w410) -> ()  [unwired: 2 in, 2 out]
          }
          frame True {
            w414 = 0 ("Top Row")
            n242 = property on="Listbox" class="LstBox (strict)"() -> ("Number of Rows"=w416:u32)  [unwired: 2 in, 2 out]
            n243 = Initialize Array(0, w416) -> (w415:i32[])
            n244 = property on="Listbox" class="LstBox (strict)"("Top Row"=w414, "Value"=w414, "Item Symbols"=w415) -> ()  [unwired: 2 in, 2 out]
          }
        }
      }
      event "Listbox": Key Down {
        n245 = event-data() -> ("VKey"=w420:T21)  [unwired: 1 in]
        n246 = case shown="\"Left\", \"Right\"" w420 {
          selector: w420 -> [w425 _]
          tunnel: eventvkey."Left" ("VKey") -> [w423 _]
          frame "Left", "Right" {
            n247 = Equal?(x=w423, y=w425) -> (x = y?=w424:bool)
            n248 = Select(t=0, s=w424, f=1) -> (s? t:f=w426:i32)
            n249 = property on="Listbox" class="LstBox (strict)"() -> ("Item Symbols"=w429:i32[])  [unwired: 2 in, 2 out]
            n250 = Replace Array Subset(array=w429, new element=w426, index="Listbox") -> (w428:i32[])
            n251 = property on="Listbox" class="LstBox (strict)"("Item Symbols"=w428) -> ()  [unwired: 2 in, 2 out]
          }
          frame Default {
          }
        }
      }
      event "DB Camera Config": Value Change {
        n252 = event-data() -> ("NewVal"=w433:bool)  [unwired: 1 in]
        n253 = case shown="False" w433 {
          tunnel: w432 -> [w442 _]
          tunnel: [w435 w453] -> w431
          tunnel: w430 -> [w434 w453]
          frame False {
            w449 = "Camera"
            w452 = FALSE ("Visible")
            n254 = local read "Camera Settings"() -> (w441:T3)
            n255 = Index Array(array=w442) -> (element=w445:cluster{string[]})  [unwired: 1 in]
            n256 = Unbundle(w441) -> ("Frate Rate"=w440:i32, "Compression"=w439:i32, "Size"=w443:u16)
            n257 = Unbundle(w445) -> (w444:string[])
            n258 = Index Array(array=w444, index=w443) -> (element=w438:string)
            n259 = call-poly <vilib>:"Write Key.vi"("section"=w449, "value"=w438, "key"="Size", "refnum"=w434) -> ("refnum out"=w451:T20)  [unwired: 2 in, 5 out]
            n260 = call-poly <vilib>:"Write Key.vi"("section"=w449, "value"=w440, "key"="FrameRate", "refnum"=w451) -> ("refnum out"=w450:T20)  [unwired: 1 in, 6 out]
            n261 = local write "DB Camera Config"(w452) -> ()
            n262 = property on="Camera Settings" class="Clust (strict)"("Visible"=w452) -> ()  [unwired: 2 in, 2 out]
            n263 = call-poly <vilib>:"Write Key.vi"("section"=w449, "value"=w439, "key"="Compression", "refnum"=w450) -> ("refnum out"=w436:T20)  [unwired: 1 in, 6 out]
            n264 = call <vilib>:"Close Config Data.vi"("refnum"=w436) -> ("file path"=w437:path)  [unwired: 2 in, 8 out]
            n265 = call <vilib>:"Open Config Data.vi"("configuration file path"=w437) -> ("refnum"=w435:T20)  [unwired: 8 in, 2 out]
          }
          frame True {
            n266 = property on="Camera Settings" class="Clust (strict)"("Visible"=TRUE) -> ()  [unwired: 2 in, 2 out]
          }
        }
      }
      event "Camera Settings": Value Change {
        n267 = event-data() -> ("NewVal"=w466:T3)  [unwired: 1 in]
        n268 = Index Array(array=w462) -> (element=w461:cluster{string[]})  [unwired: 1 in]
        n269 = Unbundle(w466) -> ("Frate Rate"=w457:i32, "Compression"=w456:i32, "Size"=w459:u16)
        n270 = Unbundle(w461) -> (w460:string[])
        n271 = Index Array(array=w460, index=w459) -> (element=w458:string)
        n272 = Format Into String(format string="%s   %dfps   %d%%", w458, w457, w456) -> (resulting string=w463:string)  [unwired: 2 in, 1 out]
        n273 = Build Array(w463) -> (w464:string[])
        n274 = property on="DB Camera Config" class="Bool (strict)"("Strings [4]"=w464) -> ()  [unwired: 2 in, 2 out]
      }
      event "Motor.Enable": Value Change {
        n275 = event-data() -> ("NewVal"=w472:bool)  [unwired: 1 in]
        n276 = Unbundle("Motor") -> ("Value"=w471:dbl)  [unwired: 1 out]
        n277 = Select(t=w471, s=w472, f=0.0) -> (s? t:f=w469:dbl)
        n278 = call <vilib>:"NT Write Number.vi"("Numeric"=w469, "Name"=w468) -> ()  [unwired: 9 in, 1 out]
      }
      event "Slider": Value Change {
        n279 = event-data() -> ("NewVal"=w475:dbl)  [unwired: 1 in]
        n280 = call <vilib>:"NT Write Number.vi"("Numeric"=w475, "Name"=w476) -> ()  [unwired: 9 in, 1 out]
      }
      event "On/Off": Value Change {
        n281 = event-data() -> ("NewVal"=w480:bool)  [unwired: 1 in]
        n282 = Boolean To (0,1)(Boolean=w480) -> (0, 1=w479:i16)
        n283 = call <vilib>:"NT Write Number.vi"("Numeric"=w479, "Name"=w478) -> ()  [unwired: 9 in, 1 out]
      }
      event "Rev/Fwd": Value Change {
        n284 = event-data() -> ("NewVal.Forward"=w488:bool, "NewVal.Reverse"=w487:bool)  [unwired: 1 in]
        n285 = Boolean To (0,1)(Boolean=w488) -> (0, 1=w484:i16)
        n286 = Boolean To (0,1)(Boolean=w487) -> (0, 1=w486:i16)
        n287 = Negate(x=w486) -> (-x=w485:i16)
        n288 = Add(x=w484, y=w485) -> (x+y=w483:i16)
        n289 = call <vilib>:"NT Write Number.vi"("Numeric"=w483, "Name"=w482) -> ()  [unwired: 9 in, 1 out]
      }
      event "Ring": Value Change {
        n290 = event-data() -> ("NewVal"=w492:u16)  [unwired: 1 in]
        n291 = property on="Ring" class="Ring (strict)"() -> ("Strings []"=w493:string[])  [unwired: 2 in, 2 out]
        n292 = Index Array(array=w493, index=w492) -> (element=w491:string)
        n293 = call <vilib>:"NT Write String.vi"("String"=w491, "Name"=w490) -> ()  [unwired: 9 in, 1 out]
      }
    }
  }
  n294 = Index Array(array=w13) -> (element=w14:cluster{string[]})  [unwired: 1 in]
  n295 = Unbundle(w14) -> (w12:string[])
  n296 = Match First String(2:w12, 3:w11) -> (0:w10:i32)  [unwired: 1 out]
  n297 = Bundle("value"=w16, "value"=w15, "index"=w10) -> (w4:cluster{"value":i32, "value":i32, "index":i32})  [unwired: 1 out]
  n298 = property on="On/Off" class="Bool (strict)"("Visible"=w27) -> ()  [unwired: 2 in, 2 out]
  n299 = property on="Motor" class="Clust (strict)"("Visible"=w27) -> ()  [unwired: 2 in, 2 out]
  n300 = property on="Progress" class="Clust (strict)"("Visible"=w27) -> ()  [unwired: 2 in, 2 out]
  n301 = property on="Ring" class="Ring (strict)"("Visible"=w27) -> ()  [unwired: 2 in, 2 out]
  n302 = property on="Rev/Fwd" class="Clust (strict)"("Visible"=w27) -> ()  [unwired: 2 in, 2 out]
  n303 = property on="Camera Settings" class="Clust (strict)"("Val(Sgnl)"=w4) -> ()  [unwired: 2 in, 2 out]
  n304 = local write "DB Camera Config"(w27) -> ()
  n305 = property on="Camera Settings" class="Clust (strict)"("Visible"=w27) -> ()  [unwired: 2 in, 2 out]
